vi "Various Globals.vi"() -> ()   [LabVIEW 2018]
panel:
  in  "Custom Elevator":dbl=5000.0
  out "Low Gear":bool=TRUE
  out "Forwards":bool=TRUE
  out "Intake Down":bool
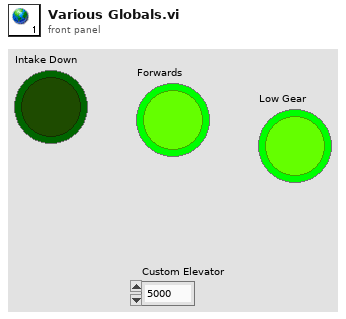
[diagram p1: front panel]
diagram:
